vi "Swerve Drive.vi"(1 "Drive Dev Ref":T1[](array[typedef]), 2 "Swerve Dev Ref":T1[](array[typedef]), 4 "X Drive":bool, 5 "error in":errorcluster, 6 "Low Sensitivity":bool, 7 "Z":dbl format="%#_13g", 8 "Reverse Drive":bool, 9 "Straight Drive":bool, 10 "Y":dbl format="%#_13g", 11 "X":dbl format="%#_13g") -> (3 "error out":errorcluster)   [LabVIEW 2016, in "Huskie Swerve.lvlib"]
uses:
  Huskie Swerve.lvlib
  <vilib>/Rock Robotics/WPI/MotorControl/WPI_MotorControlDeviceRef.ctl
  <vilib>/Rock Robotics/WPI/MotorControl/WPI_MotorControlType.ctl
  <vilib>/Rock Robotics/SystemInterfaces/DIO/FPGA_DIOPWMChannel.ctl
  <vilib>/Rock Robotics/WPI/PWM/WPI_PWMDeadband.ctl
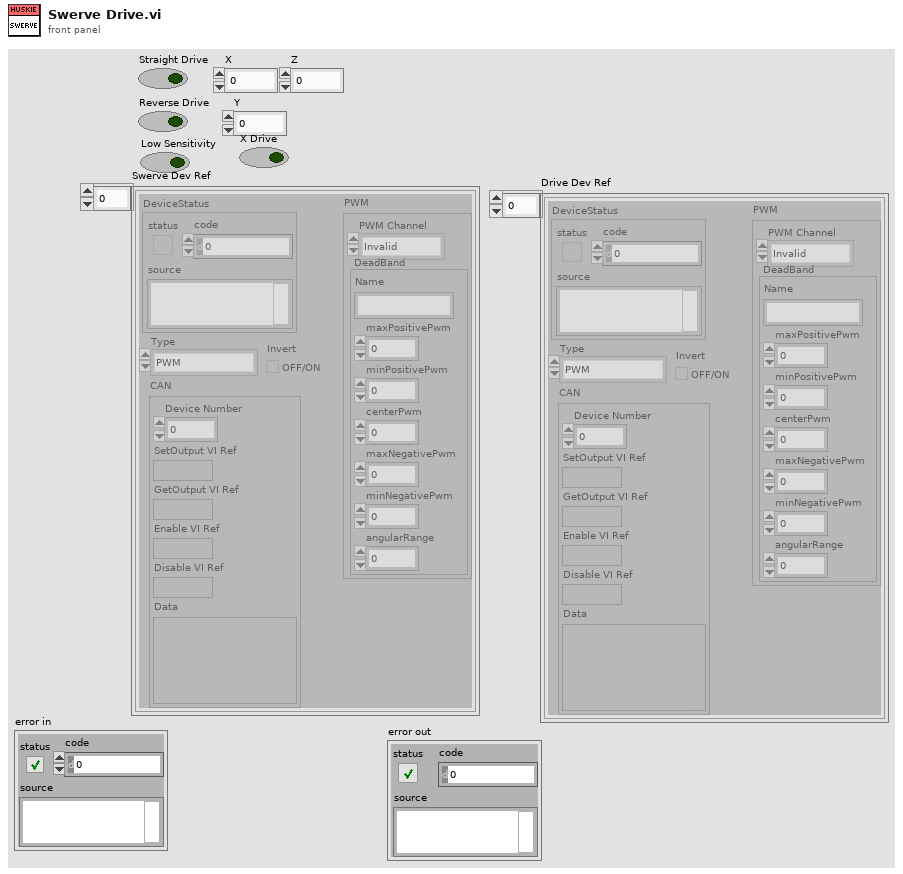
[diagram p1: front panel]
types:
  T1 = typedef "WPI_MotorControlDeviceRef.ctl" = cluster{"DeviceStatus":errorcluster, "Type":T2, "PWM":cluster{"PWM Channel":T3, "DeadBand":T4}, "CAN":cluster{"Device Number":u8, "SetOutput VI Ref":variant, "GetOutput VI Ref":variant, "Enable VI Ref":variant, "Disable VI Ref":variant, "Data":variant}, "Invert":bool}
  T2 = typedef "WPI_MotorControlType.ctl" = enum16{"PWM", "CAN"}
  T3 = typedef "FPGA_DIOPWMChannel.ctl" = enum8{"PWM 0", "PWM 1", "PWM 2", "PWM 3", "PWM 4", "PWM 5", "PWM 6", "PWM 7", "PWM 8", "PWM 9", "PWM MXP 0", "PWM MXP 1", "PWM MXP 2", "PWM MXP 3", "PWM MXP 4", "PWM MXP 5", "PWM MXP 6", "PWM MXP 7", "PWM MXP 8", "PWM MXP 9", "Invalid"}
  T4 = typedef "WPI_PWMDeadband.ctl" = cluster{"Name":string, "maxPositivePwm":i32, "minPositivePwm":i32, "centerPwm":i32, "maxNegativePwm":i32, "minNegativePwm":i32, "angularRange":u16}
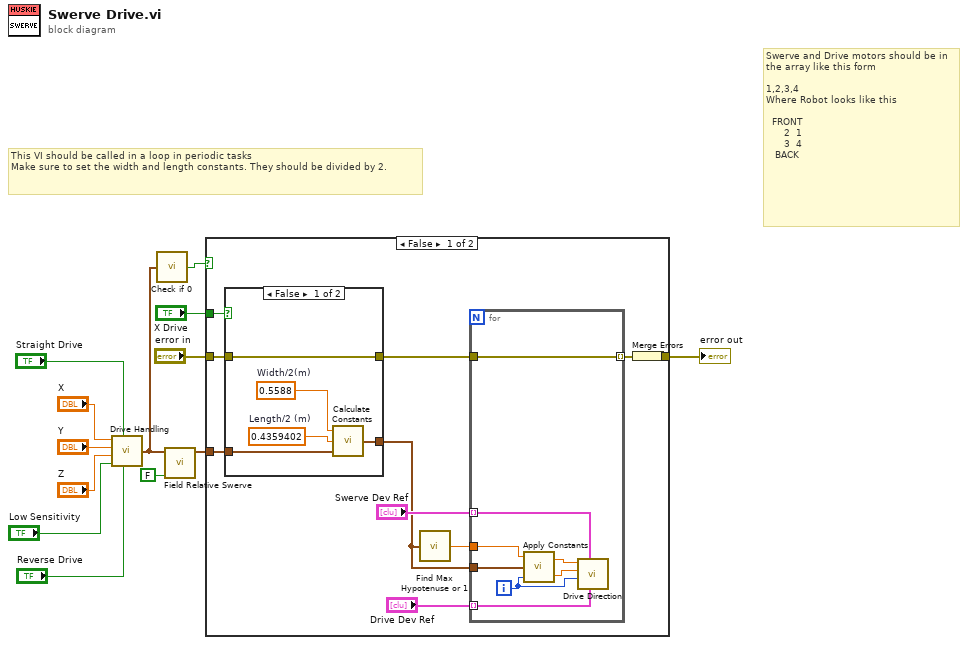
[diagram p0: block diagram]
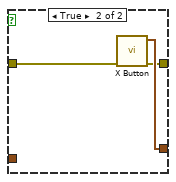
[diagram p2: hidden frame]
diagram:
  # "Swerve and Drive motors should be in the array like this form\n\n1,2,3,4\nWhere Robot looks like this\n\n  FRONT      \n      2  1\n      3  4\n   BACK"
  # "This VI should be called in a loop in periodic tasks\nMake sure to set the width and length constants. They should be divided by 2."
  n1 = call "Drive Handling.vi"("Reverse"="Reverse Drive", "Straight"="Straight Drive", "Low Sensitivity"="Low Sensitivity", "Z"="Z", "Y"="Y", "X"="X") -> ("Axes Magnitudes"=w7:cluster{"X":dbl, "Y":dbl, "Z":dbl})
  n2 = call "Check if 0.vi"("Axes Magnitudes"=w7) -> ("result"=w6:bool)
  n3 = call "Field Relative Swerve.vi"("Field Relative Active"=FALSE, "Axes Magnitudes"=w7) -> ("Axes Mag. Changed"=w2:cluster{"X":dbl, "Y":dbl, "Z":dbl})  [unwired: 9 in]
  n4 = case shown="False" w6 {
    tunnel: w2 -> [w23 _]
    tunnel: "error in" -> [w15 w40]
    tunnel: [w20 w40] -> w4
    tunnel: "X Drive" -> [w16 _]
    frame False {
      n5 = case shown="False" w16 {
        tunnel: w23 -> [w28 _]
        tunnel: [w26 w31] -> w19
        tunnel: w15 -> [w25 w30]
        tunnel: [w25 w29] -> w14
        frame False {
          w24 = 0.4359402  # Length/2 (m)
          w27 = 0.5588  # Width/2(m)
          n6 = call "Calculate Constants.vi"("Axes Magnitudes"=w28, "Length/2"=w24, "Width/2"=w27) -> ("constants cluster"=w26:cluster{"a":dbl, "b":dbl, "c":dbl, "d":dbl})
        }
        frame True {
          n7 = call "X Button.vi"("error in"=w30) -> ("error out"=w29:errorcluster, "constants cluster"=w31:cluster{"a":dbl, "b":dbl, "c":dbl, "d":dbl})  [unwired: 9 in]
        }
      }
      n8 = call "Find Max Hypotenuse or 1.vi"("constants"=w19) -> ("Max or 1"=w18:dbl)
      n9 = for {
        tunnel: w19 -> [w39]
        tunnel: w18 -> [w38]
        tunnel: "Swerve Dev Ref" -> [w35] mode=indexing
        tunnel: "Drive Dev Ref" -> [w34] mode=indexing
        tunnel: [w33] -> w17 mode=indexing
        tunnel: w14 -> [w33]
        i -> [w32]
        n10 = call "Apply Constants.vi"("Module Number"=w32, "constants cluster"=w39, "Max Speed or 1"=w38) -> ("Magnitude"=w36:dbl, "Desired Direction (rad)"=w37:dbl)
        n11 = call "Drive Direction.vi"("Drive Dev Ref"=w34, "Swerve Dev Ref"=w35, "Module Number"=w32, "Wheel Power"=w36, "Desired direction (radians)"=w37) -> ()  [unwired: 7 in]
      }
      n12 = Merge Errors(w17) -> (w20:errorcluster)
    }
    frame True {
    }
  }
  "error out" <- w4
